vi "AB_Set_Destination_Path_CORE.vi"(7 "index":i32, 8 "error in (no error)":errorcluster, 9 "new path":path, 10 "old path":path, 11 "destinations in":refnum<class "AB_Destination.lvclass">[](array[class])) -> (0 "error out":errorcluster, 3 "destinations out":refnum<class "AB_Destination.lvclass">[](array[class]))   [LabVIEW 2020]
uses:
  <vilib>/AppBuilder/AB_Classes/Destination/AB_Destination.lvclass
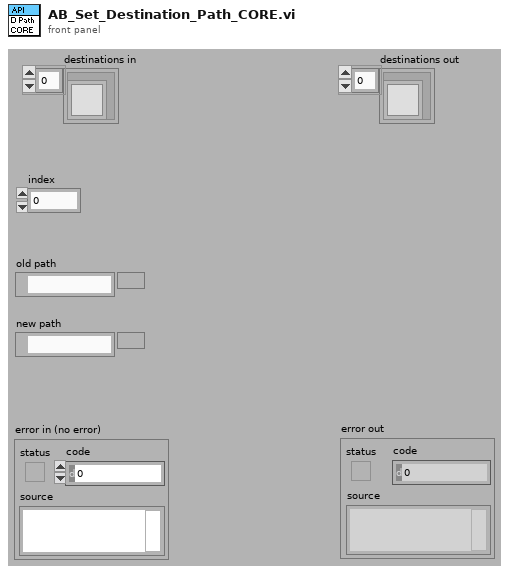
[diagram p1: front panel]
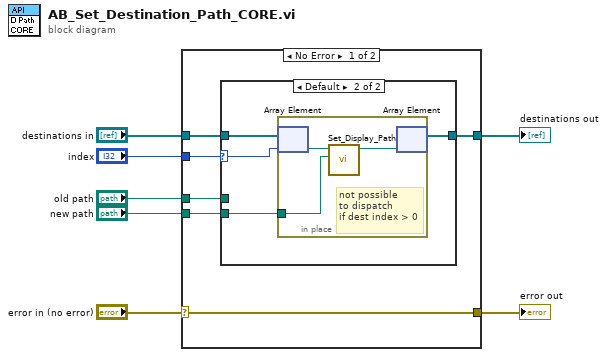
[diagram p0: block diagram]
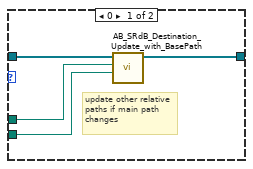
[diagram p2: hidden frame]
diagram:
  n1 = case shown="No Error" "error in (no error)" {
    selector: "error in (no error)" -> [w8 w26]
    tunnel: [w13 w25] -> w7
    tunnel: "destinations in" -> [w12 w25]
    tunnel: "new path" -> [w11 _]
    tunnel: "index" -> [w10 _]
    tunnel: "old path" -> [w9 _]
    tunnel: [w8 w26] -> w1
    frame No Error {
      n2 = case shown="Default" w10 {
        selector: w10 -> [_ w18]
        tunnel: w9 -> [w17 _]
        tunnel: w11 -> [w16 w19]
        tunnel: w12 -> [w14 w21]
        tunnel: [w15 w20] -> w13
        frame 0 {
          # "update other relative paths if main path changes"
          n3 = call <resource>:"AB_SRdB_Destination_Update_with_BasePath.vi"("new base path"=w16, "old base path"=w17, "ALL data in"=w14) -> ("ALL data out"=w15:refnum<class "AB_Destination.lvclass">[])  [unwired: 1 in, 7 out]
        }
        frame Default {
          n4 = in-place {
            in-place-border: w19 -> [w22]
            # "not possible\nto dispatch\nif dest index > 0"
            n5 = in-place-array #1(w21, w18) -> (w24:refnum<class "AB_Destination.lvclass">)
            n6 = call-dynamic "Set_Display_Path.vi"("displayPath"=w22, "AB_Destination in"=w24) -> ("AB_Destination out"=w23:refnum<class "AB_Destination.lvclass">)  [unwired: 1 in, 8 out]
            n7 = in-place-array #1(w23) -> (w20:refnum<class "AB_Destination.lvclass">[])  [unwired: 1 out]
          }
        }
      }
    }
    frame Error {
    }
  }
  "destinations out" <- w7
  "error out" <- w1
